vi "init.vi"(6 "ID query?":bool, 8 "error in (no error)":errorcluster, 9 "connect timeout ms":i32=10000, 10 "port (502)":u16=502, 11 "address":string) -> (0 "error out":errorcluster, 2 "ID string":string, 3 "Modbus Master out":refnum<class "Modbus Master.lvclass">)   [LabVIEW 2018]
uses:
  <vilib>/NI/Modbus Library/API/Master/Modbus Master.lvclass
  <vilib>/NI/Modbus Library/API/Wrapper/Create TCP Master.vi
  <vilib>/NI/Modbus Library/API/Wrapper/API Main.lvlib
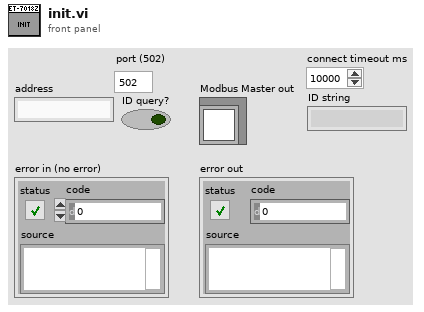
[diagram p1: front panel]
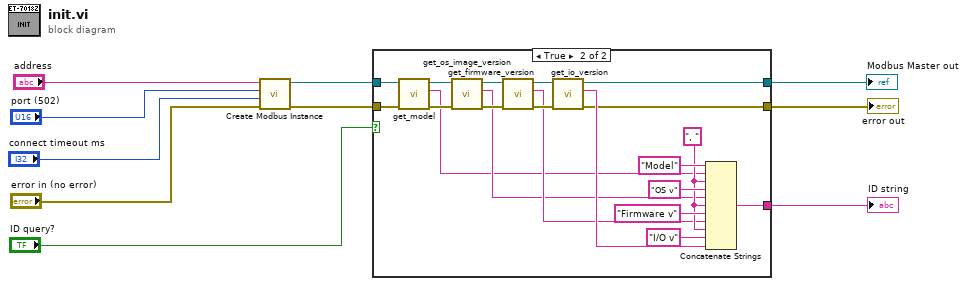
[diagram p0: block diagram]
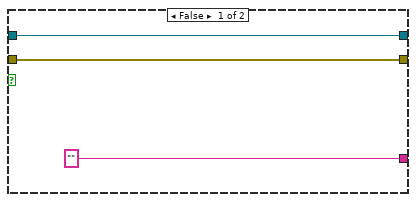
[diagram p2: hidden frame]
diagram:
  n1 = call-poly <vilib>:"Create Modbus Instance.vi"("error in"="error in (no error)", "connect timeout ms"="connect timeout ms", "port (502)"="port (502)", "address"="address") -> ("error out"=w4:errorcluster, "TCP master instance"=w6:refnum<class "Modbus Master.lvclass">)  [unwired: 6 in]
  n2 = case shown="True" "ID query?" {
    tunnel: w6 -> [w13 w18]
    tunnel: [w13 w20] -> w5
    tunnel: w4 -> [w12 w17]
    tunnel: [w12 w19] -> w3
    tunnel: ["" w21] -> w1
    frame False {
    }
    frame True {
      w25 = ", " ("string")
      n3 = call "get_model.vi"("error in (no error)"=w17, "Modbus Master in"=w18) -> ("error out"=w16:errorcluster, "Model"=w14:string, "Modbus Master out"=w15:refnum<class "Modbus Master.lvclass">)  [unwired: 7 in]
      n4 = call "get_os_image_version.vi"("error in (no error)"=w16, "Modbus Master in"=w15) -> ("error out"=w32:errorcluster, "OS image version"=w22:string, "Modbus Master out"=w33:refnum<class "Modbus Master.lvclass">)  [unwired: 7 in]
      n5 = call "get_firmware_version.vi"("error in (no error)"=w32, "Modbus Master in"=w33) -> ("error out"=w30:errorcluster, "Firmware version"=w23:string, "Modbus Master out"=w31:refnum<class "Modbus Master.lvclass">)  [unwired: 7 in]
      n6 = call "get_io_version.vi"("error in (no error)"=w30, "Modbus Master in"=w31) -> ("error out"=w19:errorcluster, "I/O version"=w24:string, "Modbus Master out"=w20:refnum<class "Modbus Master.lvclass">)  [unwired: 7 in]
      n7 = Concatenate Strings("Model" ("string"), w14, w25, "OS v" ("string"), w22, w25, "Firmware v" ("string"), w23, w25, "I/O v" ("string"), w24) -> (w21:string)
    }
  }
  "error out" <- w3
  "Modbus Master out" <- w5
  "ID string" <- w1
